vi "Sort Array In Reverse.vi"(0 "InputArray":string[](array[string]), 11 "error in (no error)":errorcluster) -> (4 "SortedArray":string[](array[string]), 15 "error out":errorcluster)   [LabVIEW 2021, in "CustomSortPath.lvlib"]
doc: "This Vi gets the input string array and gives out the sorted string array in reverse order."
uses:
  CustomSortPath.lvlib
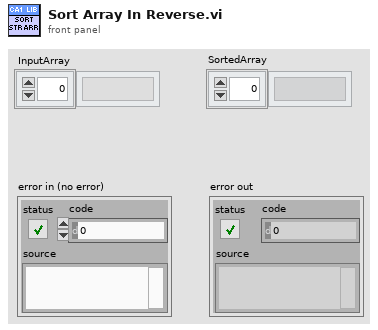
[diagram p1: front panel]
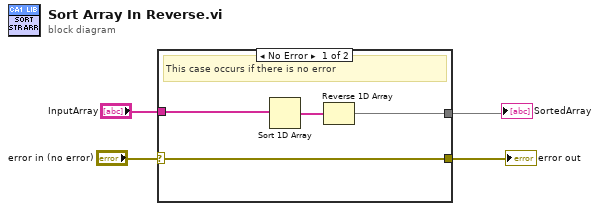
[diagram p0: block diagram]
diagram:
  n1 = case shown="No Error" "error in (no error)" {
    selector: "error in (no error)" -> [w7 w9]
    tunnel: [w7 w9] -> w3
    tunnel: [w6 _] -> w2
    tunnel: "InputArray" -> [w5 _]
    frame No Error {
      # "This case occurs if there is no error"
      n2 = Sort 1D Array(array=w5) -> (sorted array=w8:string[])
      n3 = Reverse 1D Array(array=w8) -> (reversed array=w6:string[])
    }
    frame Error {
      # "This case occurs if there is any error."
    }
  }
  "error out" <- w3
  "SortedArray" <- w2
